vi "get_duration.vi"(8 "error in (no error)":errorcluster, 11 "ImagingModeDL090130Frame in":refnum<class "ImagingModeDL090130Frame.lvclass">=refnum) -> (0 "error out":errorcluster, 2 "duration":dbl[unit], 3 "ImagingModeDL090130Frame out":refnum<class "ImagingModeDL090130Frame.lvclass">)   [LabVIEW 2010, in "ImagingModeDL090130Frame.lvclass"]
uses:
  ImagingModeDL090130Frame.lvclass
  ImagingModeDL090130Frame.lvclass/ImagingModeDL090130Frame.ctl
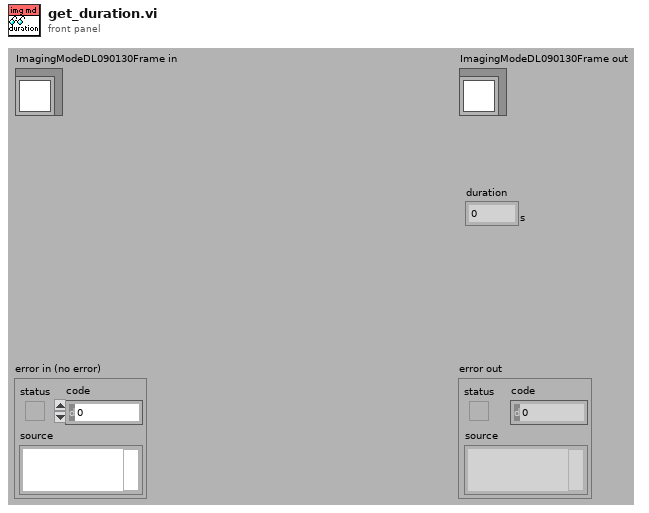
[diagram p1: front panel]
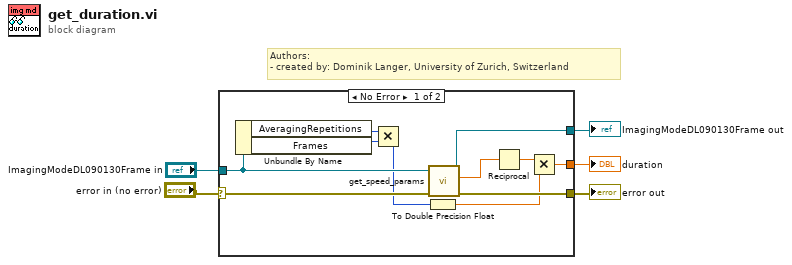
[diagram p0: block diagram]
diagram:
  # "Authors: \n- created by: Dominik Langer, University of Zurich, Switzerland"
  n1 = case shown="No Error" "error in (no error)" {
    selector: "error in (no error)" -> [w9 w18]
    tunnel: [w16 w18] -> w4
    tunnel: [w15 w17] -> w2
    tunnel: "ImagingModeDL090130Frame in" -> [w12 w17]
    tunnel: [w13 _] -> w1
    frame No Error {
      n2 = Unbundle By Name(w12) -> ("AveragingRepetitions"=w8:i32, "Frames"=w7:i32)
      n3 = Multiply(x=w8, y=w7) -> (x*y=w6:i32)
      n4 = To Double Precision Float(number=w6) -> (double precision float=w10:dbl)
      n5 = call-dynamic "get_speed_params.vi"("error in (no error)"=w9, "ImagingModeDL090130Frame in"=w12) -> ("error out"=w16:errorcluster, "frame rate"=w14:dbl[unit], "ImagingModeDL090130Frame out"=w15:refnum<class "ImagingModeDL090130Frame.lvclass">)  [unwired: 4 in, 3 out]
      n6 = Reciprocal(x=w14) -> (1/x=w11:dbl[unit])
      n7 = Multiply(x=w11, y=w10) -> (x*y=w13:dbl[unit])
    }
    frame Error {
    }
  }
  "error out" <- w4
  "ImagingModeDL090130Frame out" <- w2
  "duration" <- w1
